vi "tempSensor.vi"() -> ()   [LabVIEW 2023]
uses:
  <vilib>/DAQmx/read.llb/DAQmx Read (Analog DBL 1Chan 1Samp).vi
  <vilib>/DAQmx/read.llb/DAQmx Read (Analog Wfm 1Chan 1Samp).vi
  <vilib>/DAQmx/create/channels.llb/DAQmx Create Channel (AI-Temperature-Thermocouple).vi
  <vilib>/DAQmx/configure/timing.llb/DAQmx Timing (Sample Clock).vi
  <vilib>/DAQmx/miscellaneous.llb/DAQmx Fill In Error Info.vi
  <vilib>/Waveform/WDTOps.llb/WDT Get Waveform Time Array DBL.vi
panel:
  out "Waveform Chart":dbl(graph)
  in  "thermocouple type":i32(ring)=10072 items=["J"=10072, "K"=10073, "N"=10077, "R"=10082, "S"=10085, "T"=10086, "B"=10047, "E"=10055]
  out "temp":dbl
  in  "Record":bool
  in  "Save location":string
  in  "Save as":string
  in  "Sample rate (Hz)":dbl=1000.0 format="%0.2f"
  in  "?":bool
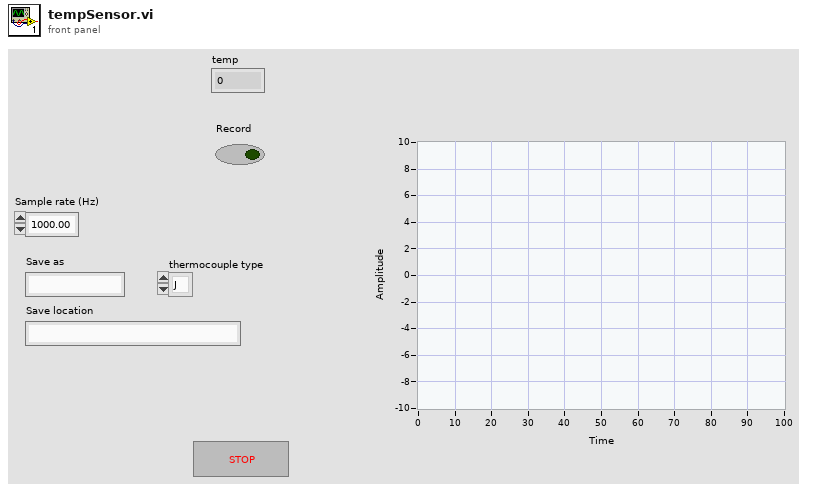
[diagram p1: front panel]
types:
  T1 = enum16{"open", "open or create", "create or replace", "create", "open (read-only)"}
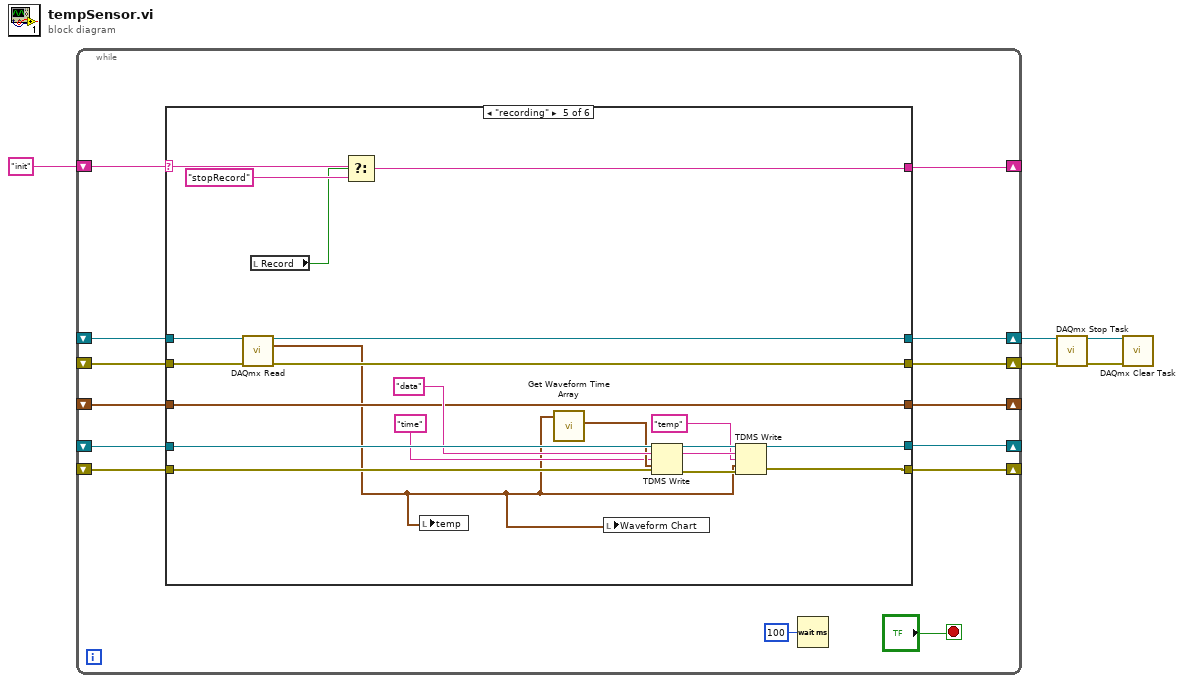
[diagram p0: block diagram]
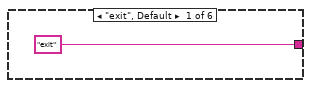
[diagram p2: hidden frame]
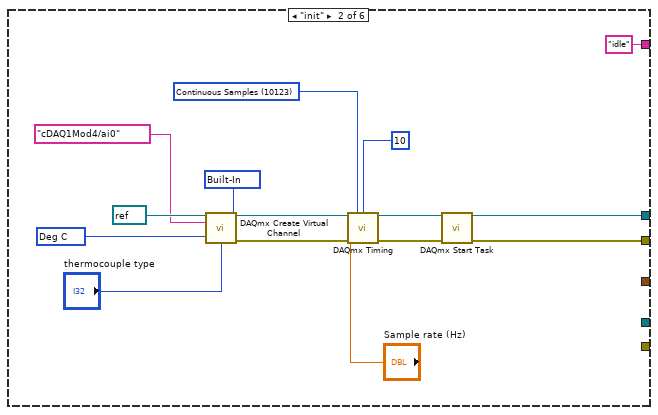
[diagram p3: hidden frame]
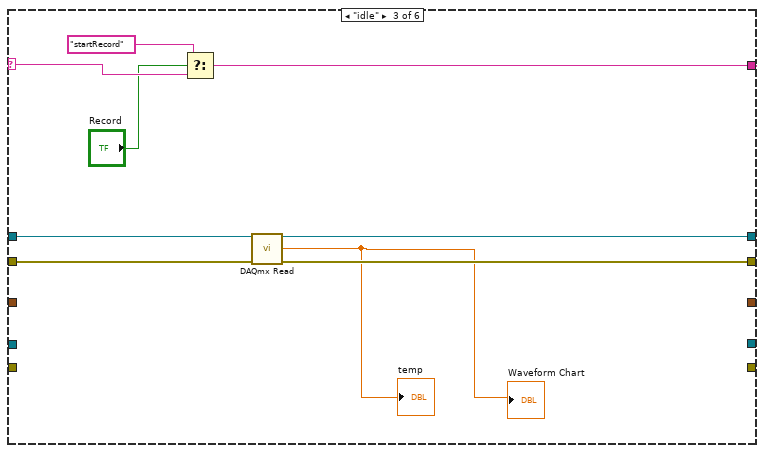
[diagram p4: hidden frame]
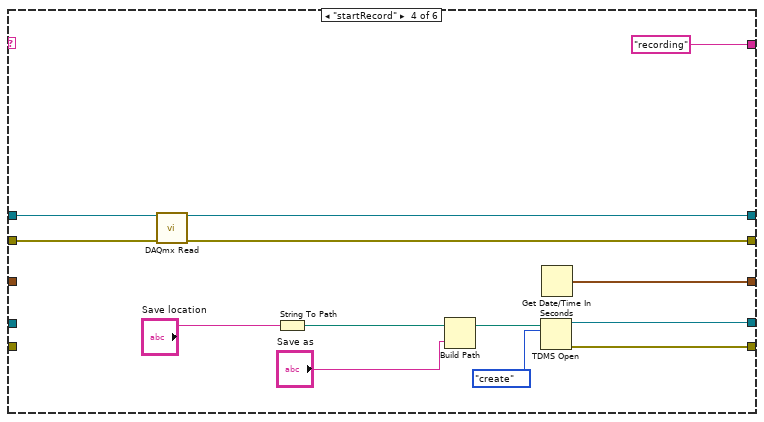
[diagram p5: hidden frame]
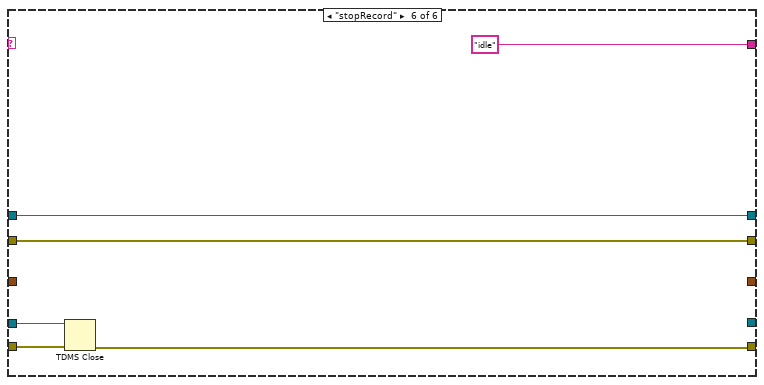
[diagram p6: hidden frame]
diagram:
  n1 = while {
    shift-right: [w17] -> _
    shift-left: "init" -> [w18]
    shift-right: [w15] -> w4
    shift-left: _ -> [w14]
    shift-right: [w16] -> w3
    shift-left: _ -> [w13]
    shift-right: [w9] -> _
    shift-left: _ -> [w6]
    shift-right: [w10] -> _
    shift-left: _ -> [w8]
    shift-right: [w11] -> _
    shift-left: _ -> [w7]
    stop <- "?" stop-if-true
    n2 = case shown="\"recording\"" w18 {
      selector: w18 -> [_ _ w44 _ w78 _]
      tunnel: ["exit" "idle" ("f") w42 "recording" w76 "idle"] -> w17
      tunnel: [_ w34 w37 w53 w73 w82] -> w16
      tunnel: [_ w31 w38 w54 w72 w83] -> w15
      tunnel: w14 -> [_ _ w40 w56 w75 w83]
      tunnel: w13 -> [_ _ w39 w55 w74 w82]
      tunnel: [_ _ _ w47 w63 w79] -> w11
      tunnel: [_ _ _ w46 w65 _] -> w10
      tunnel: [_ _ _ w45 w68 _] -> w9
      tunnel: w8 -> [_ _ _ _ w71 w81]
      tunnel: w7 -> [_ _ _ _ w70 w80]
      tunnel: w6 -> [_ _ _ _ w68 _]
      frame "exit", Default {
      }
      frame "init" {
        w24 = 10143 items=["Deg C"=10143, "Deg F"=10144, "Kelvins"=10325, "Deg R"=10145, "From Custom Scale"=10065] ("units")
        w25 = 10200 items=["Built-In"=10200, "Constant Value"=10116, "Channel"=10113] ("cjc source")
        w26 = 10123 items=["Finite Samples"=10178, "Continuous Samples"=10123, "Hardware Timed Single Point"=12522] ("sample mode")
        n3 = call-poly <vilib>:"DAQmx Create Virtual Channel.vi"("task in"=refnum<k21> refnum, "physical channels"=tag "cDAQ1Mod4/ai0", "cjc source"=w25, "units"=w24, "thermocouple type"="thermocouple type") -> ("task out"=w29:refnum<k21>, "error out"=w28:errorcluster)  [unwired: 9 in]
        n4 = call-poly <vilib>:"DAQmx Timing.vi"("task/channels in"=w29, "sample mode"=w26, "samples per channel"=10, "rate"="Sample rate (Hz)", "error in"=w28) -> ("task out"=w33:refnum<k21>, "error out"=w35:errorcluster)  [unwired: 9 in]
        n5 = call <vilib>:"DAQmx Start Task.vi"("task/channels in"=w33, "error in"=w35) -> ("task out"=w31:refnum<k21>, "error out"=w34:errorcluster)  [unwired: 12 in]
      }
      frame "idle" {
        n6 = Select(t="startRecord", s="Record", f=w44) -> (s? t:f=w42:string)
        n7 = call-poly <vilib>:"DAQmx Read.vi"("task/channels in"=w40, "error in"=w39) -> ("task out"=w38:refnum<k21>, "data"=→"temp" →"Waveform Chart":dbl, "error out"=w37:errorcluster)  [unwired: 11 in]
      }
      frame "startRecord" {
        n8 = call-poly <vilib>:"DAQmx Read.vi"("task/channels in"=w56, "error in"=w55) -> ("task out"=w54:refnum<k21>, "error out"=w53:errorcluster)  [unwired: 11 in, 1 out]
        n9 = String To Path(string="Save location") -> (path=w51:path)
        n10 = Build Path(base path=w51, name or relative path="Save as") -> (appended path=w48:path)
        n11 = TDMS Open(10:T1."create" ("operation (0:open)"), 11:w48) -> (0:w47:errorcluster, 3:w46:refnum<k34>)  [unwired: 5 in]
        n12 = Get Date/Time In Seconds() -> (seconds since 1Jan1904=w45:timestamp)
      }
      frame "recording" {
        n13 = call-poly <vilib>:"DAQmx Read.vi"("task/channels in"=w75, "error in"=w74) -> ("task out"=w72:refnum<k21>, "data"=w58:waveform(dbl), "error out"=w73:errorcluster)  [unwired: 11 in]
        n14 = local read "Record"() -> (w67:bool)
        n15 = Select(t=w78, s=w67, f="stopRecord") -> (s? t:f=w76:string)
        n16 = local write "temp"(w58) -> ()
        n17 = call-poly <vilib>:"Get Waveform Time Array.vi"("waveform in"=w58) -> ("X array"=w60:timestamp[])  [unwired: 9 in, 1 out]
        n18 = local write "Waveform Chart"(w58) -> ()
        n19 = TDMS Write(0:w71, 5:"data", 7:"time", 9:w60, 11:w70) -> (4:w66:refnum<k34>, 6:w62:string, 15:w64:errorcluster)  [unwired: 1 in, 1 out]
        n20 = TDMS Write(0:w66, 5:w62, 7:"temp", 9:w58, 11:w64) -> (4:w65:refnum<k34>, 15:w63:errorcluster)  [unwired: 1 in, 2 out]
      }
      frame "stopRecord" {
        n21 = TDMS Close(8:w80, 11:w81) -> (0:w79:errorcluster)  [unwired: 1 out]
      }
    }
    n22 = Wait (ms)(milliseconds to wait=u32 100) -> ()  [unwired: 1 out]
  }
  n23 = call <vilib>:"DAQmx Stop Task.vi"("task/channels in"=w4, "error in"=w3) -> ("task out"=w2:refnum<k21>, "error out"=w1:errorcluster)  [unwired: 12 in]
  n24 = call <vilib>:"DAQmx Clear Task.vi"("task in"=w2, "error in"=w1) -> ()  [unwired: 13 in, 1 out]
